vi "New Main.vi"() -> ()   [LabVIEW 2021]
uses:
  <vilib>/Platform/TimedLoop/XDataNode/timing_clust.ctl
  <vilib>/Platform/TimedLoop/XDataNode/nitl_modes.ctl
  <vilib>/Platform/TimedLoop/XDataNode/wakeup.ctl
  <vilib>/platform/TimedLoop/XDataNode/XDataNode.xnode
  <vilib>/Platform/TimedLoop/XDataNode/XDNodeRunTimeDep.lvlib
panel:
  out "Waveform Graph":waveform(dbl)[](graph)
  in  "Analog Input Mode":enum16{"High Accuracy", "High Speed"}(ring)
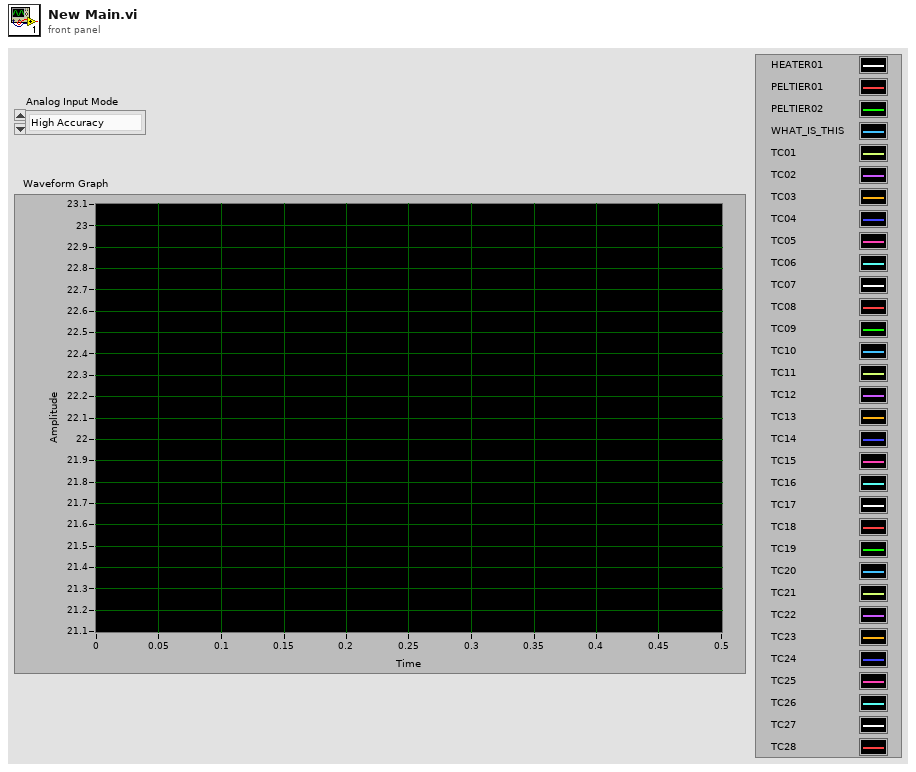
[diagram p1: front panel]
types:
  T1 = typedef "XDNodeRunTimeDep.lvlib/timing_clust.ctl" = cluster{"Expected End [f-1]":u64, "Actual End [f-1]":u64, "Finished Late? [f-1]":bool, "Expected End [i-1]":u64, "Actual End [i-1]":u64, "Finished Late? [i-1]":bool, "Expected Start [i]":u64, "Actual Start [i]":u64, "Expected Start [f]":u64, "Actual Start [f]":u64, "Source Name":string, "Structure Name":string, "Period":i64, "Deadline":i64, "Offset":i64, "Start":i64, "Priority":i32, "Timeout":i32, "Mode":T2, "Wakeup Reason":T3, "Error":errorcluster, "Source Type":string, "Secondary Source Type":string, "Global End Time":u64, "Global Start Time":u64, "Frame Duration":u64, "Iteration Duration":u64, "Assigned CPU":i32, "I/O Scan Engine Mode":u32}
  T2 = typedef "XDNodeRunTimeDep.lvlib/nitl_modes.ctl" = enum32{"No Change", "Process missed periods, maintain original phase", "Discard missed periods, maintain original phase", "Process missed periods, ignore original phase", "Discard missed periods, ignore original phase"}
  T3 = typedef "XDNodeRunTimeDep.lvlib/wakeup.ctl" = enum32{"Normal", "Aborted", "Asynchronous wakeup", "Timing source error", "Timed loop error", "Timeout"}
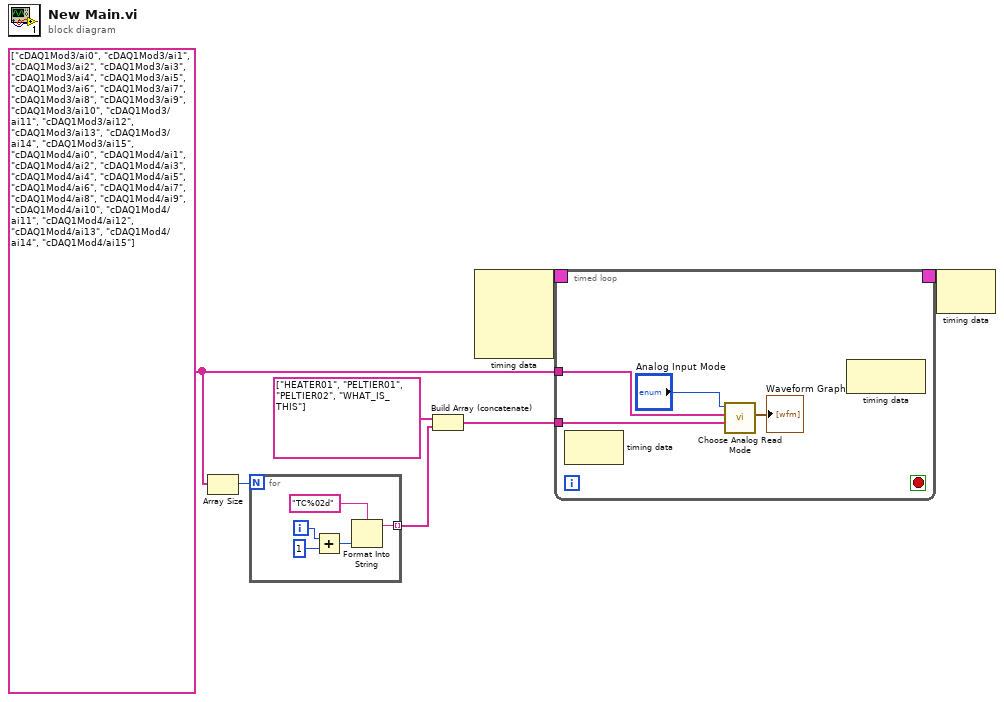
[diagram p0: block diagram]
diagram:
  w7 = tag[] ["cDAQ1Mod3/ai0", "cDAQ1Mod3/ai1", "cDAQ1Mod3/ai2", "cDAQ1Mod3/ai3", "cDAQ1Mod3/ai4", "cDAQ1Mod3/ai5", "cDAQ1Mod3/ai6", "cDAQ1Mod3/ai7", "cDAQ1Mod3/ai8", "cDAQ1Mod3/ai9", "cDAQ1Mod3/ai10", "cDAQ1Mod3/ai11", "cDAQ1Mod3/ai12", "cDAQ1Mod3/ai13", "cDAQ1Mod3/ai14", "cDAQ1Mod3/ai15", "cDAQ1Mod4/ai0", "cDAQ1Mod4/ai1", "cDAQ1Mod4/ai2", "cDAQ1Mod4/ai3", "cDAQ1Mod4/ai4", "cDAQ1Mod4/ai5", "cDAQ1Mod4/ai6", "cDAQ1Mod4/ai7", "cDAQ1Mod4/ai8", "cDAQ1Mod4/ai9", "cDAQ1Mod4/ai10", "cDAQ1Mod4/ai11", "cDAQ1Mod4/ai12", "cDAQ1Mod4/ai13", "cDAQ1Mod4/ai14", "cDAQ1Mod4/ai15"]
  n1 = Array Size(array=w7) -> (size(s)=w6:i32)
  n2 = for {
    N: w6 -> [_]
    tunnel: [w11] -> w5 mode=indexing
    i -> [w10]
    n3 = Add(x=w10, y=1) -> (x+y=w9:i32)
    n4 = Format Into String(format string="TC%02d", w9) -> (resulting string=w11:string)  [unwired: 2 in, 1 out]
  }
  n5 = Build Array (concatenate)(string[] ["HEATER01", "PELTIER01", "PELTIER02", "WHAT_IS_THIS"], w5) -> (w3:string[])
  n6 = node-c288() -> (w2:T1)  [unwired: 4 in]
  n7 = timed-loop {
    timing: w2 -> [_]
    timing-out: [_] -> w1
    tunnel: w7 -> [w16]
    tunnel: w3 -> [w15]
    stop <- _ stop-if-true
    n8 = node-c288() -> ()  [unwired: 1 in, 1 out]
    n9 = call "Choose Analog Read Mode.vi"("Channel Names"=w15, "Physical Channels"=w16, "Analog Input Mode"="Analog Input Mode") -> ("data"=→"Waveform Graph":waveform(dbl)[])  [unwired: 8 in]
    n10 = node-c288() -> ()  [unwired: 1 in, 1 out]
  }
  n11 = node-c288(w1) -> ()  [unwired: 1 out]
